vi "Drive Straight.vi"(6 "Encoder Gain - Slow":dbl, 8 "Sensitivity":dbl=1.0, 9 "Distance":dbl, 10 "Speed":dbl, 11 "Encoder Gain - Fast":dbl) -> (2 "At Distance":bool)   [LabVIEW 2013]
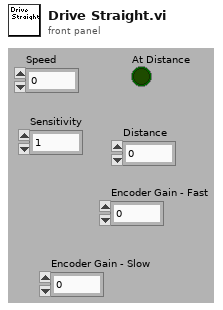
[diagram p1: front panel]
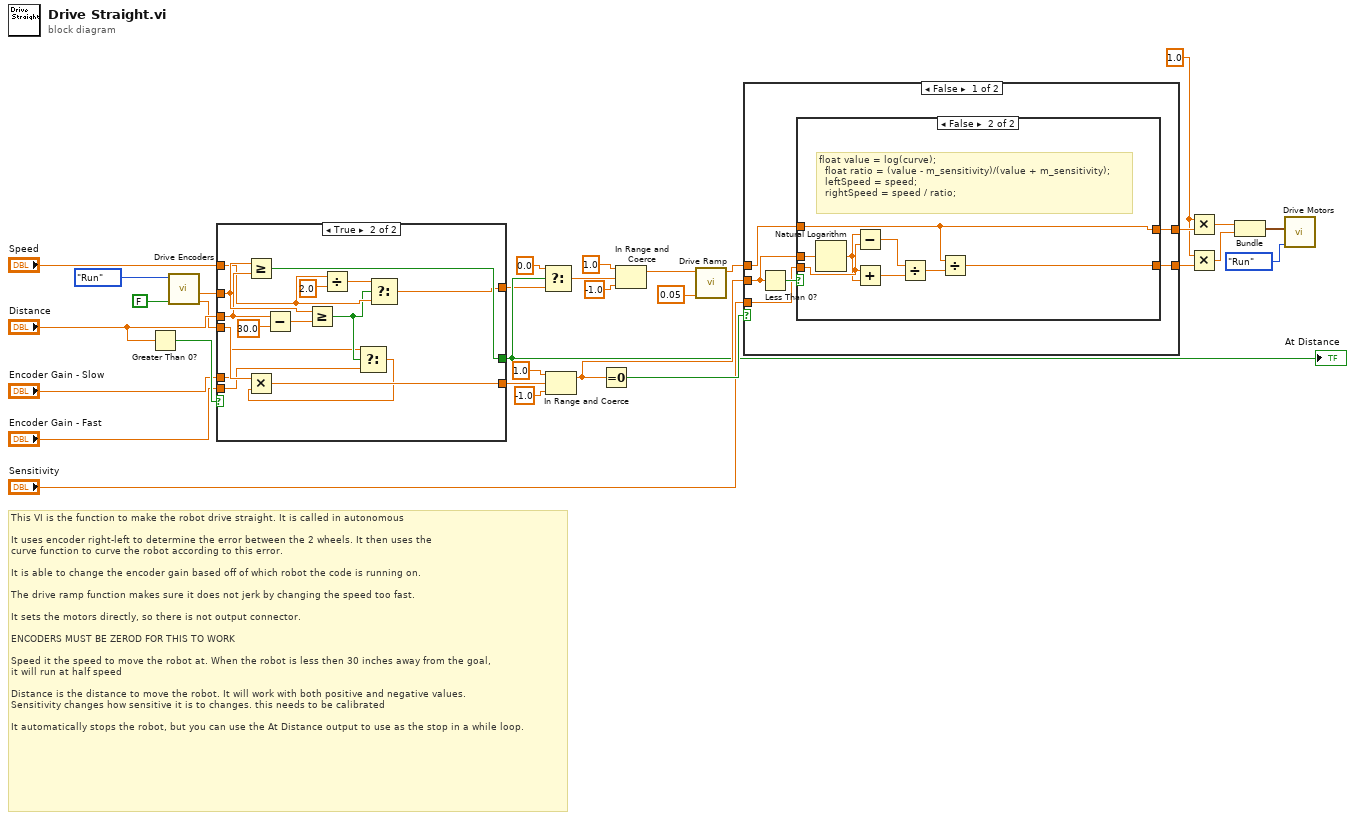
[diagram p0: block diagram]
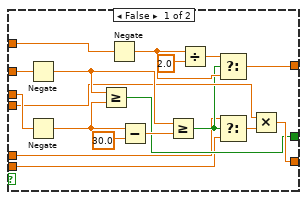
[diagram p2: hidden frame]
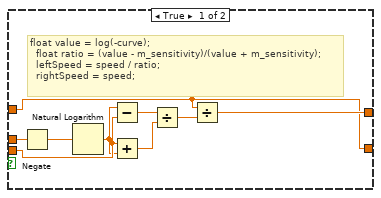
[diagram p3: hidden frame]
diagram:
  w22 = 1.0
  # "This VI is the function to make the robot drive straight. It is called in autonomous\n\nIt uses encoder right-left to determine the error between the 2 wheels. It then uses the\ncurve function to curve the robot according to this error.\n\nIt is able to change the encoder gain based off of which robot the code is running on.\n\nThe drive ramp function makes sure it does not jerk by changing the speed too fast.\n\nIt sets the motors directly, so there is not output connector.\n\nENCODERS MUST BE ZEROD FOR THIS TO WORK\n\nSpeed it the speed to move the robot at. When the robot is less then 30 inches away from the goal,\nit will run at half speed\n\nDistance is the distance to move the robot. It will work with both positive and negative values.\nSensitivity changes how sensitive it is to changes. this needs to be calibrated\n\nIt automatically stops the robot, but you can use the At Distance output to use as the stop in a while loop."
  n1 = Greater Than 0?(x="Distance") -> (x > 0?=w20:bool)
  n2 = call "Drive Encoders.vi"("Reset Encoders?"=FALSE, "Mode"=enum16{"Init", "Run", "End"}."Run") -> ("Right-Left"=w9:dbl, "Average Distance"=w15:dbl)  [unwired: 2 in, 6 out]
  n3 = case shown="True" w20 {
    tunnel: [w49 w64] -> w10
    tunnel: w15 -> [w40 w62]
    tunnel: "Distance" -> [w41 w60]
    tunnel: [w44 w63] -> w14
    tunnel: "Speed" -> [w38 w56]
    tunnel: [w43 w55] -> w12
    tunnel: w9 -> [w36 w54]
    tunnel: "Encoder Gain - Fast" -> [w33 w51]
    tunnel: "Encoder Gain - Slow" -> [w34 w50]
    frame False {
      n4 = Negate(x=w40) -> (-x=w39:dbl)
      n5 = Negate(x=w41) -> (-x=w42:dbl)
      n6 = Greater Or Equal?(x=w39, y=w42) -> (x >= y?=w44:bool)
      n7 = Negate(x=w38) -> (-x=w37:dbl)
      n8 = Subtract(x=w42, y=30.0) -> (x-y=w45:dbl)
      n9 = Greater Or Equal?(x=w39, y=w45) -> (x >= y?=w35:bool)
      n10 = Divide(x=w37, y=2.0) -> (x/y=w48:dbl)
      n11 = Select(t=w48, s=w35, f=w37) -> (s? t:f=w43:dbl)
      n12 = Select(t=w34, s=w35, f=w33) -> (s? t:f=w32:dbl)
      n13 = Multiply(x=w36, y=w32) -> (x*y=w49:dbl)
    }
    frame True {
      n14 = Greater Or Equal?(x=w62, y=w60) -> (x >= y?=w63:bool)
      n15 = Subtract(x=w60, y=30.0) -> (x-y=w61:dbl)
      n16 = Greater Or Equal?(x=w62, y=w61) -> (x >= y?=w53:bool)
      n17 = Divide(x=w56, y=2.0) -> (x/y=w57:dbl)
      n18 = Select(t=w50, s=w53, f=w51) -> (s? t:f=w52:dbl)
      n19 = Multiply(x=w54, y=w52) -> (x*y=w64:dbl)
      n20 = Select(t=w57, s=w53, f=w56) -> (s? t:f=w55:dbl)
    }
  }
  "At Distance" <- w14
  n21 = Select(t=0.0, s=w14, f=w12) -> (s? t:f=w11:dbl)
  n22 = In Range and Coerce(upper limit=1.0, x=w10, lower limit=-1.0) -> (coerced(x)=w24:dbl)  [unwired: 1 out]
  n23 = Equal To 0?(x=w24) -> (x = 0?=w31:bool)
  n24 = In Range and Coerce(upper limit=1.0, x=w11, lower limit=-1.0) -> (coerced(x)=w3:dbl)  [unwired: 1 out]
  n25 = call "Drive Ramp.vi"("Max Delta Per Iteration"=0.05, "Input"=w3) -> ("Output"=w4:dbl)  [unwired: 9 out]
  n26 = case shown="False" w31 {
    tunnel: w4 -> [w69 w88]
    tunnel: [w66 w88] -> w30
    tunnel: [w65 w88] -> w29
    tunnel: w24 -> [w68 _]
    tunnel: "Sensitivity" -> [w67 _]
    frame False {
      n27 = Less Than 0?(x=w68) -> (x < 0?=w70:bool)
      n28 = case shown="False" w70 {
        tunnel: w67 -> [w76 w87]
        tunnel: w68 -> [w77 w86]
        tunnel: w69 -> [w72 w82]
        tunnel: [w73 w82] -> w66
        tunnel: [w72 w80] -> w65
        frame True {
          # "float value = log(-curve);\n\t\tfloat ratio = (value - m_sensitivity)/(value + m_sensitivity);\n\t\tleftSpeed = speed / ratio;\n\t\trightSpeed = speed;"
          n29 = Negate(x=w77) -> (-x=w75:dbl)
          n30 = Natural Logarithm(1:w75) -> (0:w71:dbl)
          n31 = Subtract(x=w71, y=w76) -> (x-y=w79:dbl)
          n32 = Add(x=w76, y=w71) -> (x+y=w78:dbl)
          n33 = Divide(x=w79, y=w78) -> (x/y=w74:dbl)
          n34 = Divide(x=w72, y=w74) -> (x/y=w73:dbl)
        }
        frame False {
          # "float value = log(curve);\n\t\tfloat ratio = (value - m_sensitivity)/(value + m_sensitivity);\n\t\tleftSpeed = speed;\n\t\trightSpeed = speed / ratio;"
          n35 = Natural Logarithm(1:w86) -> (0:w85:dbl)
          n36 = Subtract(x=w85, y=w87) -> (x-y=w84:dbl)
          n37 = Add(x=w87, y=w85) -> (x+y=w83:dbl)
          n38 = Divide(x=w84, y=w83) -> (x/y=w81:dbl)
          n39 = Divide(x=w82, y=w81) -> (x/y=w80:dbl)
        }
      }
    }
    frame True {
    }
  }
  n40 = Multiply(x=w22, y=w30) -> (x*y=w8:dbl)
  n41 = Multiply(x=w22, y=w29) -> (x*y=w7:dbl)
  n42 = Bundle(w8, w7) -> (w6:cluster{dbl, dbl})  [unwired: 1 out]
  n43 = call "Drive Motors.vi"("Mode"=enum16{"Init", "Run", "End"}."Run", "Inputs"=w6) -> ()  [unwired: 2 in, 8 out]
